vi "Climber Controller.vi"(8 "error in":errorcluster) -> ()   [LabVIEW 2017]
doc: "This VI executes continuously carrying out the current operation and responding to updates or new operations. It will often contain the timing or control code that is difficult to place directly in TeleOp. This VI generally opens all sensors and motors and isolates the rest of the robot code from knowing how the operations are carried out."
uses:
  Climber Setpoints.ctl
  Climber Operations.ctl
  Users/Public/Documents/Cross The Road Electronics/Phoenix-LabVIEW/Motor Controller/Controls/CTRE_Phoenix_MotorControl_ControlMode.ctl
  <vilib>/Rock Robotics/WPI/ThirdParty/Phoenix-LabVIEW/Motor Controller/Controls/CTRE_Phoenix_MotorControl_NeutralMode.ctl
  <vilib>/Rock Robotics/WPI/Solenoid/WPI_SolenoidChannel.ctl
  <vilib>/Rock Robotics/WPI/Solenoid/WPI_SolenoidValue.ctl
  <vilib>/Rock Robotics/WPI/Solenoid/WPI_SolenoidOpenSingle.vi
  <vilib>/Rock Robotics/WPI/Solenoid/WPI_SolenoidSetEnum.vi
  <vilib>/Rock Robotics/Network Tables/NT Write Boolean.vi
panel:
  out "Current\nCmd":string
  # "Tip: It may be helpful to observe inputs and sensor values.\nYou may also want to display tuning or debugging controls."
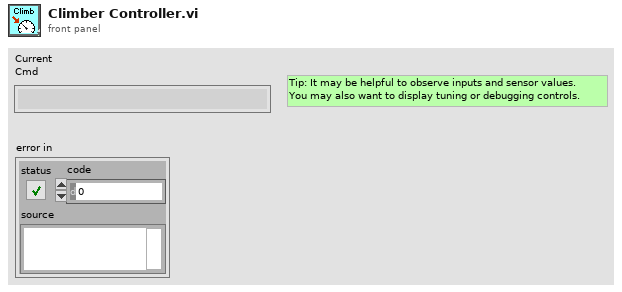
[diagram p1: front panel]
types:
  T1 = typedef "WPI_SolenoidValue.ctl" = enum16{"Off", "On", "Forward", "Reverse"}
  T2 = typedef "WPI_SolenoidChannel.ctl" = enum8{"Solenoid 0", "Solenoid 1", "Solenoid 2", "Solenoid 3", "Solenoid 4", "Solenoid 5", "Solenoid 6", "Solenoid 7", "Invalid"}
  T3 = typedef "CTRE_Phoenix_MotorControl_NeutralMode.ctl" = enum8{"EEPROMSetting", "Override to Coast", "Override to Brake"}
  T4 = typedef "CTRE_Phoenix_MotorControl_ControlMode.ctl" = u16
  T5 = typedef "Climber Setpoints.ctl" = cluster{"Operation":T6, "Climber Speed":dbl, "Duration":dbl}
  T6 = typedef "Climber Operations.ctl" = enum16{"Reserve", "Read Current", "Climb", "Climber Out", "Climber In"}
  T7 = typedef "WPI_MotorControlDeviceRef.ctl" = cluster{"DeviceStatus":errorcluster, "Type":T8, "PWM":cluster{"PWM Channel":T9, "DeadBand":T10}, "CAN":cluster{"Device Number":u8, "SetOutput VI Ref":variant, "GetOutput VI Ref":variant, "Enable VI Ref":variant, "Disable VI Ref":variant, "Data":variant}, "Invert":bool, "DIO PWM":cluster{"PWM \"Enable\" Channel":T9, "DIOChannel":T11, "PWM Rate":dbl}}
  T8 = typedef "WPI_MotorControlType.ctl" = enum16{"PWM", "CAN", "DIO PWM"}
  T9 = typedef "FPGA_DIOPWMChannel.ctl" = enum8{"PWM 0", "PWM 1", "PWM 2", "PWM 3", "PWM 4", "PWM 5", "PWM 6", "PWM 7", "PWM 8", "PWM 9", "PWM MXP 0", "PWM MXP 1", "PWM MXP 2", "PWM MXP 3", "PWM MXP 4", "PWM MXP 5", "PWM MXP 6", "PWM MXP 7", "PWM MXP 8", "PWM MXP 9", "Invalid"}
  T10 = typedef "WPI_PWMDeadband.ctl" = cluster{"Name":string, "maxPositivePwm":i32, "minPositivePwm":i32, "centerPwm":i32, "maxNegativePwm":i32, "minNegativePwm":i32, "angularRange":u16}
  T11 = typedef "FPGA_DIOChannel.ctl" = enum8{"DIO 0", "DIO 1", "DIO 2", "DIO 3", "DIO 4", "DIO 5", "DIO 6", "DIO 7", "DIO 8", "DIO 9", "DIO MXP 0", "DIO MXP 1", "DIO MXP 2", "DIO MXP 3", "DIO MXP 4", "DIO MXP 5", "DIO MXP 6", "DIO MXP 7", "DIO MXP 8", "DIO MXP 9", "DIO MXP 10", "DIO MXP 11", "DIO MXP 12", "DIO MXP 13", "DIO MXP 14", "DIO MXP 15", "SPI Port CS1", "SPI Port CS2", "SPI Port CS3", "SPI Port MISO", "SPI Port MOSI", "Invalid"}
  T12 = typedef "WPI_SolenoidDevRef.ctl" = cluster{"DevStatus":errorcluster, "Pneumatics Control Module":u8, "Forward Solenoid Channel":T2, "Reverse Solenoid Channel":T2}
  T13 = typedef "Command Status Info.ctl" = cluster{"Name":string, "Status":T14, "notifier out":T15}
  T14 = typedef "Completion Status.ctl" = enum16{"Successful", "Aborted", "Incomplete"}
  T15 = typedef "Completion Notifier.ctl" = refnum<notifier>
  T16 = cluster{"Default Command":T5, "Command Timing":cluster{"Start Time (ms)":u32, "Iterations":i32}, "Command Arguments":cluster{"Command Info":T13, "Description":string, "Default Command":T5, "notifier out":refnum<notifier>, "Subsystem Name":string}}
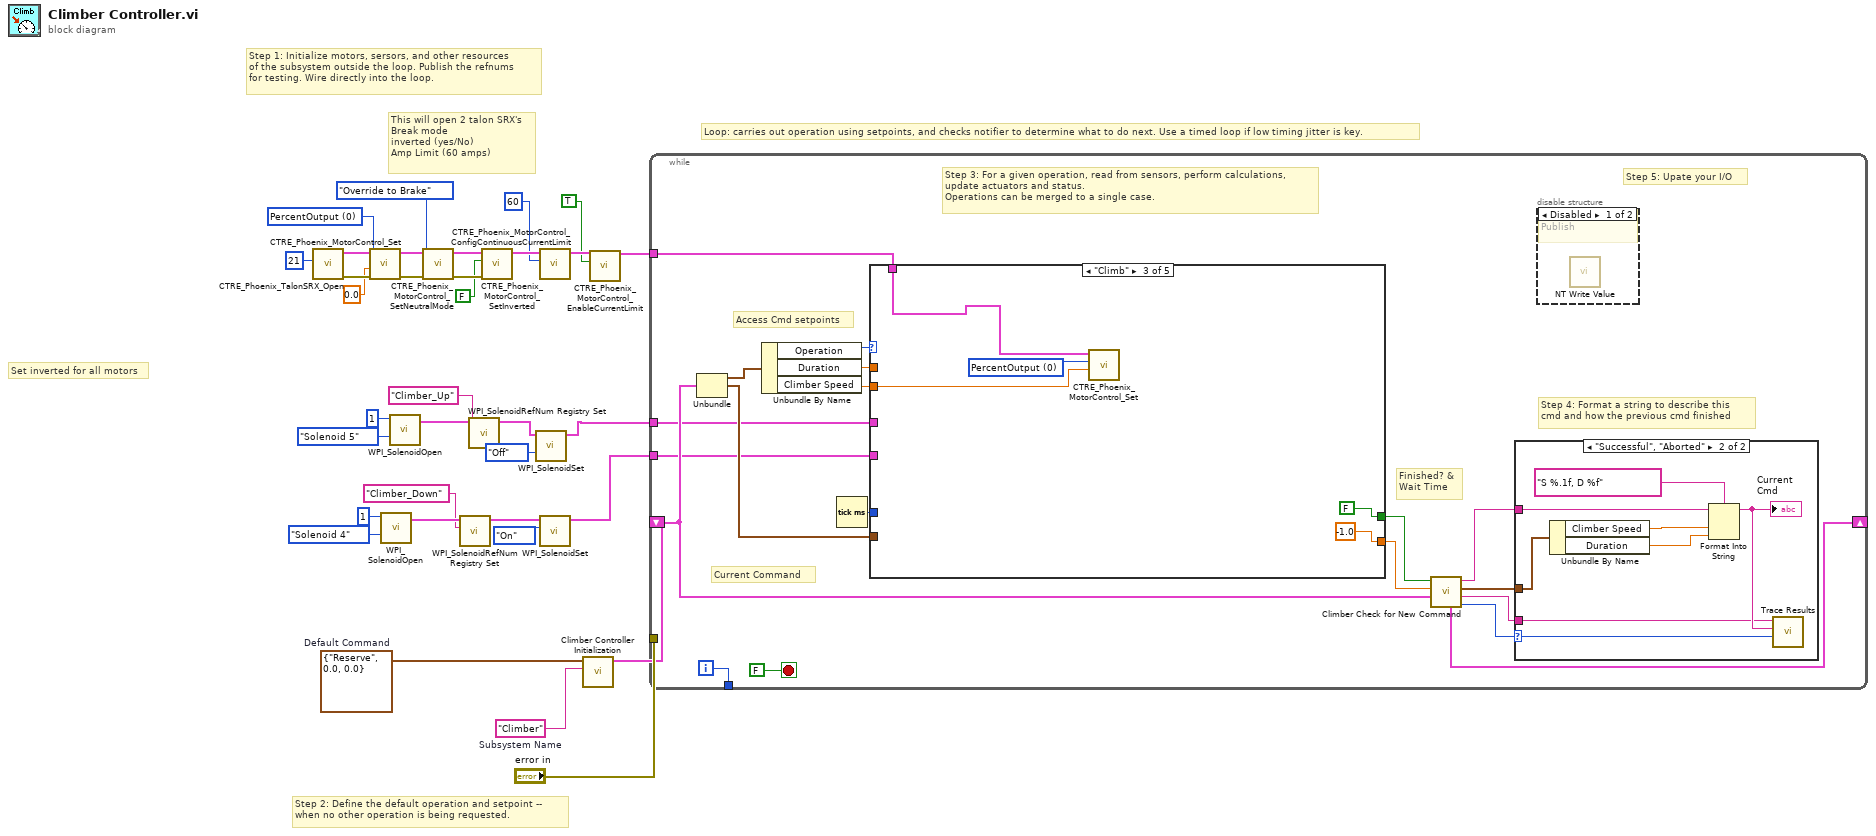
[diagram p0: block diagram]
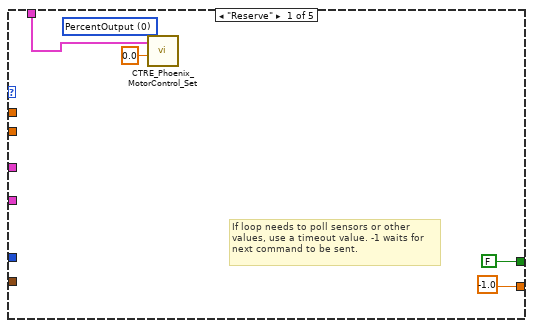
[diagram p4: hidden frame]
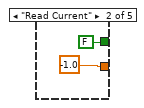
[diagram p5: hidden frame]
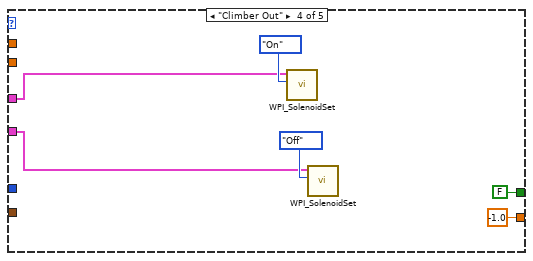
[diagram p6: hidden frame]
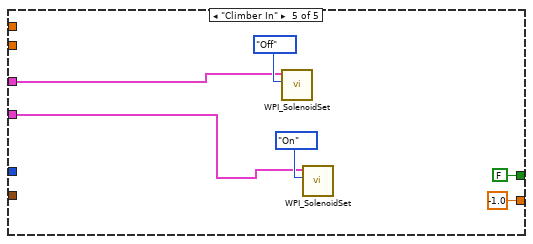
[diagram p7: hidden frame]
diagram:
  w28 = T4 0 items=["PercentOutput"=0, "Position"=1, "Velocity"=2, "Follower"=5, "MotionProfile"=6, "MotionMagic"=7, "MotionMagicArc"=8, "TimedPercentOutput"=9, "Disabled"=15] ("Control Mode")
  w31 = T5 {"Operation"=enum."Reserve", "Climber Speed"=0.0, "Duration"=0.0}  # Default Command
  w32 = "Climber"  # Subsystem Name
  # "This will open 2 talon SRX's\nBreak mode\ninverted (yes/No)\nAmp Limit (60 amps)"
  # "Set inverted for all motors"
  # "Step 2: Define the default operation and setpoint --\nwhen no other operation is being requested."
  # "Step 1: Initialize motors, sersors, and other resources\nof the subsystem outside the loop. Publish the refnums\nfor testing. Wire directly into the loop."
  # "Loop: carries out operation using setpoints, and checks notifier to determine what to do next. Use a timed loop if low timing jitter is key."
  n1 = call <vilib>:"CTRE_Phoenix_TalonSRX_Open.vi"("Device Number"=u8 21) -> ("error out"=w30:errorcluster, "CAN Talon SRX Ref"=w29:T7)  [unwired: 9 in]
  n2 = call <vilib>:"CTRE_Phoenix_MotorControl_Set.vi"("error in (no error)"=w30, "Output"=0.0, "Control Mode"=w28, "PhoenixMotorControlDevRef"=w29) -> ("error out"=w25:errorcluster, "PhoenixMotorControlDevRef"=w24:T7)  [unwired: 6 in]
  n3 = call-poly <vilib>:"WPI_SolenoidOpen.vi"("Solenoid Channel"=WPI_SolenoidChannel."Solenoid 4", "Pneumatics Control Module (0)"=u8 1) -> ("SolenoidDevRef"=w10:T12)  [unwired: 8 in, 1 out]
  n4 = call-poly <vilib>:"WPI_SolenoidOpen.vi"("Solenoid Channel"=WPI_SolenoidChannel."Solenoid 5", "Pneumatics Control Module (0)"=u8 1) -> ("SolenoidDevRef"=w14:T12)  [unwired: 8 in, 1 out]
  n5 = call <vilib>:"CTRE_Phoenix_MotorControl_SetNeutralMode.vi"("error in (no error)"=w25, "Motor Control Neutral Mode"=CTRE_Phoenix_MotorControl_NeutralMode."Override to Brake", "PhoenixMotorControlDevRef"=w24) -> ("error out"=w22:errorcluster, "PhoenixMotorControlDevRef"=w21:T7)  [unwired: 7 in]
  n6 = call <vilib>:"WPI_SolenoidRefNum Registry Set.vi"("refnum name"="Climber_Down", "SolenoidDevRef"=w10) -> ("SolenoidDevRef"=w2:T12)  [unwired: 8 in, 1 out]
  n7 = call <vilib>:"WPI_SolenoidRefNum Registry Set.vi"("refnum name"="Climber_Up", "SolenoidDevRef"=w14) -> ("SolenoidDevRef"=w6:T12)  [unwired: 8 in, 1 out]
  n8 = call <vilib>:"CTRE_Phoenix_MotorControl_SetInverted.vi"("error in (no error)"=w22, "Invert?"=FALSE, "PhoenixMotorControlDevRef"=w21) -> ("PhoenixMotorControlDevRef"=w19:T7)  [unwired: 7 in, 1 out]
  n9 = call-poly <vilib>:"WPI_SolenoidSet.vi"("Value"=WPI_SolenoidValue."Off", "SolenoidDevRef"=w6) -> ("SolenoidDevRef"=w4:T12)  [unwired: 8 in, 1 out]
  n10 = call <vilib>:"CTRE_Phoenix_MotorControl_ConfigContinuousCurrentLimit.vi"("Continuous Current Limit (Amps)"=60, "PhoenixMotorControlDevRef"=w19) -> ("PhoenixMotorControlDevRef"=w17:T7)  [unwired: 8 in, 1 out]
  n11 = call-poly <vilib>:"WPI_SolenoidSet.vi"("Value"=WPI_SolenoidValue."On", "SolenoidDevRef"=w2) -> ("SolenoidDevRef"=w3:T12)  [unwired: 8 in, 1 out]
  n12 = call "Climber Controller Initialization.vi"("Subsystem Name"=w32, "Default Command"=w31) -> ("Command Info"=w33:T16)  [unwired: 9 in]
  n13 = call <vilib>:"CTRE_Phoenix_MotorControl_EnableCurrentLimit.vi"("Enable Current Limit?"=TRUE, "PhoenixMotorControlDevRef"=w17) -> ("PhoenixMotorControlDevRef"=w15:T7)  [unwired: 8 in, 1 out]
  n14 = while {
    shift-right: [w44] -> _
    shift-left: w33 -> [w45]
    tunnel: [w52] -> _
    tunnel: "error in" -> [_]
    tunnel: w15 -> [w37]
    tunnel: w4 -> [w36]
    tunnel: w3 -> [w35]
    i -> [w52]
    stop <- FALSE stop-if-true
    # "Step 5: Upate your I/O"
    # "Step 4: Format a string to describe this\ncmd and how the previous cmd finished"
    # "Current Command"
    # "Access Cmd setpoints"
    # "Finished? &\nWait Time"
    # "Step 3: For a given operation, read from sensors, perform calculations,\nupdate actuators and status.\nOperations can be merged to a single case."
    n15 = Unbundle(w45) -> ("Default Command"=w51:T5, "Command Timing"=w47:cluster{"Start Time (ms)":u32, "Iterations":i32})  [unwired: 1 out]
    n16 = Unbundle By Name(w51) -> ("Operation"=w50:T6, "Duration"=w49:dbl, "Climber Speed"=w46:dbl)
    n17 = Tick Count (ms)() -> (millisecond timer value=w48:u32)
    n18 = case shown="\"Climb\"" w50 {
      tunnel: [-1.0 -1.0 -1.0 -1.0 -1.0] -> w42
      tunnel: [FALSE ("ignore previous (F)") FALSE ("ignore previous (F)") FALSE ("ignore previous (F)") FALSE ("ignore previous (F)") FALSE ("ignore previous (F)")] -> w43
      tunnel: w47 -> [_ _ _ _ _]
      tunnel: w49 -> [_ _ _ _ _]
      tunnel: w48 -> [_ _ _ _ _]
      tunnel: w46 -> [_ _ w69 _ _]
      tunnel: w37 -> [w62 _ w70 _ _]
      tunnel: w36 -> [_ _ _ w75 w83]
      tunnel: w35 -> [_ _ _ w74 w82]
      frame "Reserve" {
        w64 = T4 0 items=["PercentOutput"=0, "Position"=1, "Velocity"=2, "Current"=3, "Follower"=5, "MotionProfile"=6, "MotionMagic"=7, "MotionMagicArc"=8, "MotionProfileArc"=10, "Disabled"=15] ("Control Mode")
        # "If loop needs to poll sensors or other\nvalues, use a timeout value. -1 waits for\nnext command to be sent."
        n19 = call <vilib>:"CTRE_Phoenix_MotorControl_Set.vi"("Output"=0.0, "Control Mode"=w64, "PhoenixMotorControlDevRef"=w62) -> ()  [unwired: 7 in, 2 out]
      }
      frame "Read Current" {
      }
      frame "Climb" {
        w71 = T4 0 items=["PercentOutput"=0, "Position"=1, "Velocity"=2, "Current"=3, "Follower"=5, "MotionProfile"=6, "MotionMagic"=7, "MotionMagicArc"=8, "MotionProfileArc"=10, "Disabled"=15] ("Control Mode")
        n20 = call <vilib>:"CTRE_Phoenix_MotorControl_Set.vi"("Output"=w69, "Control Mode"=w71, "PhoenixMotorControlDevRef"=w70) -> ()  [unwired: 7 in, 2 out]
      }
      frame "Climber Out" {
        n21 = call-poly <vilib>:"WPI_SolenoidSet.vi"("Value"=WPI_SolenoidValue."On", "SolenoidDevRef"=w75) -> ()  [unwired: 8 in, 2 out]
        n22 = call-poly <vilib>:"WPI_SolenoidSet.vi"("Value"=WPI_SolenoidValue."Off", "SolenoidDevRef"=w74) -> ()  [unwired: 8 in, 2 out]
      }
      frame "Climber In" {
        n23 = call-poly <vilib>:"WPI_SolenoidSet.vi"("Value"=WPI_SolenoidValue."Off", "SolenoidDevRef"=w83) -> ()  [unwired: 8 in, 2 out]
        n24 = call-poly <vilib>:"WPI_SolenoidSet.vi"("Value"=WPI_SolenoidValue."On", "SolenoidDevRef"=w82) -> ()  [unwired: 8 in, 2 out]
      }
    }
    n25 = call "Climber Check for New Command.vi"("Current Command"=w45, "Wait time (ms)"=w42, "Finished?"=w43) -> ("Completion"=w38:T14, "Subsystem Name"=w39:string, "Current Command"=w40:T5, "Initial Trace String"=w41:string, "NextCommand"=w44:T16)  [unwired: 4 in]
    n26 = case shown="\"Successful\", \"Aborted\"" w38 {
      selector: w38 -> [_ w61]
      tunnel: w41 -> [_ w57]
      tunnel: w40 -> [_ w58]
      tunnel: w39 -> [_ w54]
      frame "Incomplete", Default {
        # "Continuing current command"
      }
      frame "Successful", "Aborted" {
        # "Report and setup for next command"
        n27 = Unbundle By Name(w58) -> ("Climber Speed"=w60:dbl, "Duration"=w55:dbl)
        n28 = Format Into String(format string="S %.1f, D %f", initial string=w57, w60, w55) -> (resulting string=w56:string)  [unwired: 1 in, 1 out]
        "Current\nCmd" <- w56
        n29 = call <vilib>:"Trace Results.vi"("Status of previous command"=w61, "Description"=w56, "Subsystem"=w54) -> ()  [unwired: 9 in]
      }
    }
    n30 = disable-structure shown="Disabled" {
      frame Disabled {
        # "Publish"
        n31 = call-poly <vilib>:"NT Write Value.vi"() -> ()  [unwired: 11 in, 1 out]
      }
      frame Enabled {
      }
    }
  }
